vi "Write TCP Network Connection Refnum.vi"(8 "error in (no error)":errorcluster, 10 "TCP Network Connection Refnum":refnum<k5>, 11 "TCPCommunicator in":refnum<class "TCPCommunicator.lvclass">) -> (0 "error out":errorcluster, 3 "TCPCommunicator out":refnum<class "TCPCommunicator.lvclass">)   [LabVIEW 2016, in "TCPCommunicator.lvclass"]
uses:
  TCPCommunicator.lvclass
  TCPCommunicator.lvclass/TCPCommunicator.ctl
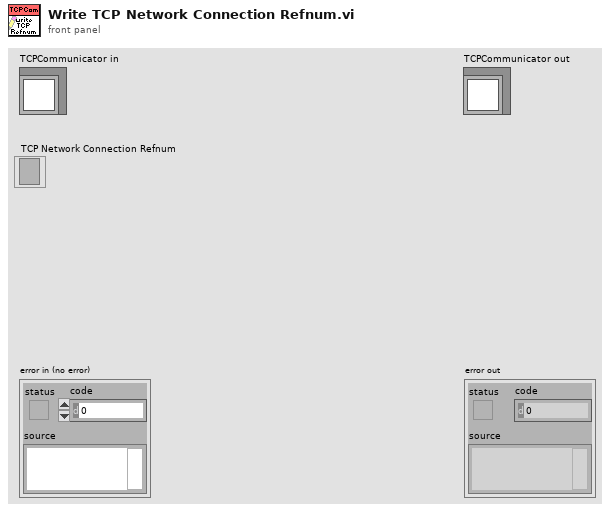
[diagram p1: front panel]
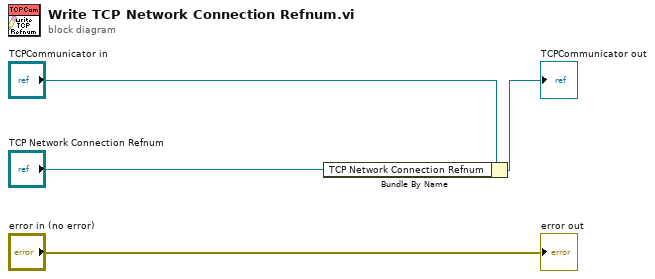
[diagram p0: block diagram]
diagram:
  n1 = Bundle By Name(cluster="TCPCommunicator in", "TCP Network Connection Refnum"="TCP Network Connection Refnum") -> (→"TCPCommunicator out":refnum<class "TCPCommunicator.lvclass">)
  "error out" <- "error in (no error)"
